vi "WAV_u16.vi"(9 "data string":string, 10 "u16":u16, 11 "String in":string) -> (3 "String out":string)   [LabVIEW 2022 SP3]
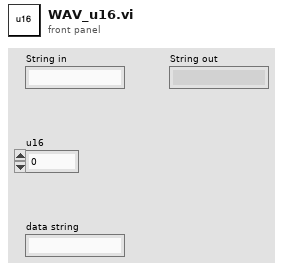
[diagram p1: front panel]
types:
  T1 = enum16{"big-endian, network order", "native, host order", "little-endian"}
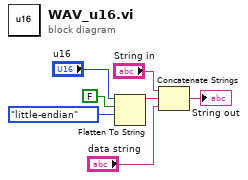
[diagram p0: block diagram]
diagram:
  n1 = Flatten To String(anything="u16", prepend array or string size? (T)=FALSE, byte order (0:big-endian, network order)=T1."little-endian") -> (data string=w6:string)  [unwired: 1 in, 2 out]
  n2 = Concatenate Strings("String in", w6, "data string") -> (→"String out":string)
